vi "emi_Set Application version from Constant.vi"(0 "VI with revision number(this vI)":refnum<vi>, 7 "Version Info in":T1={"Name"="Default Name", "Major"=0, "Minor"=0, "Fix"=0, "Build"=0, "Type"=enum."Alfa", "Dev"=FALSE, "Version Name"="", "Date"=timestamp(0 s since 1904-01-01)} {"Date" format="%<%y%m%d>T"}, 11 "error in (no error)":errorcluster) -> (4 "VI Refnum Out":refnum<vi>, 15 "error out":errorcluster)   [LabVIEW 2011]
doc: "Set the application version information from constant.\n\nWill try to update build and date(on build updated) on version constant on calling diagram\n\nOn error. Sett version anyway, asuming directly from constant. Wil not set version info"
uses:
  Private/emi_Version Info.ctl
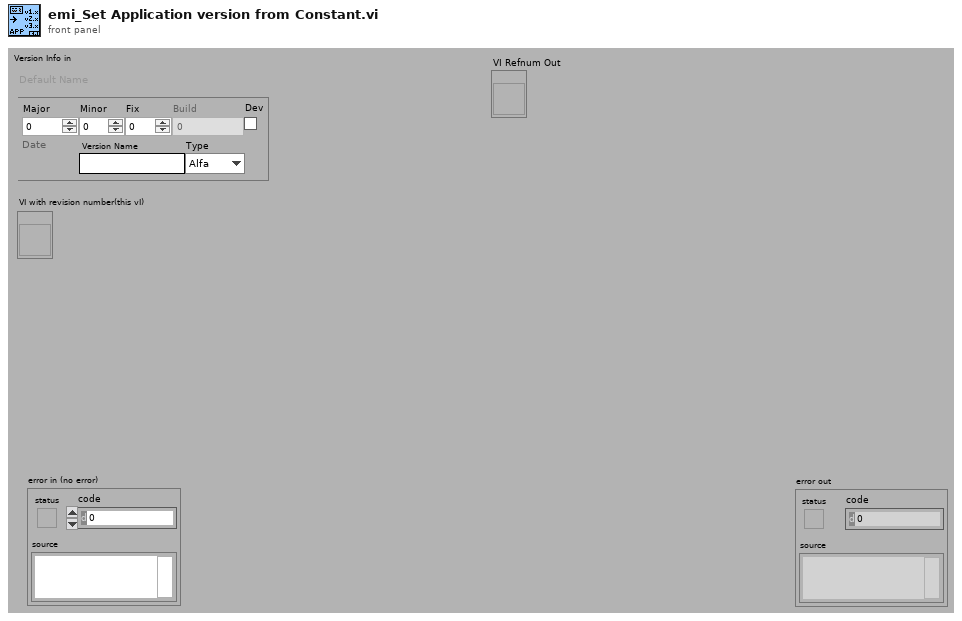
[diagram p1: front panel]
types:
  T1 = typedef "emi_Version Info.ctl" = cluster{"Name":string, "Major":i16, "Minor":i16, "Fix":i16, "Build":i32, "Type":enum16{"Alfa", "Beta", "Stable"}, "Dev":bool, "Version Name":string, "Date":timestamp}
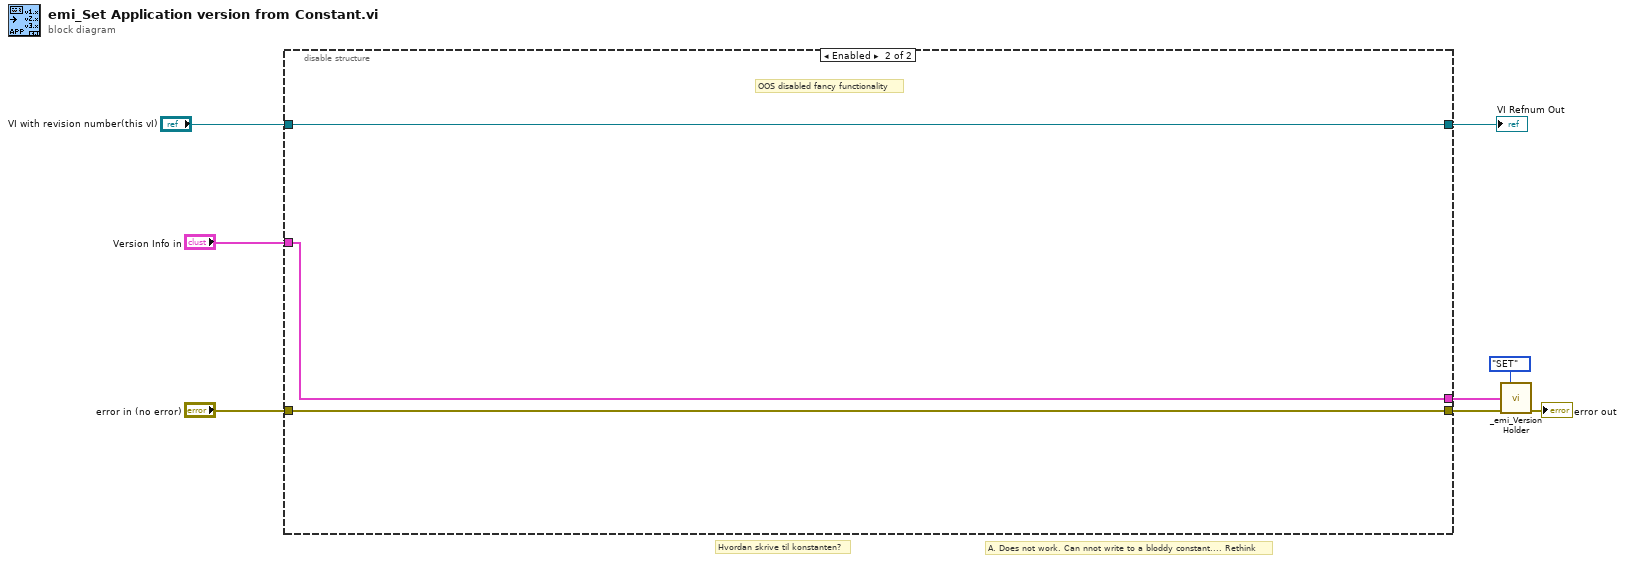
[diagram p0: block diagram]
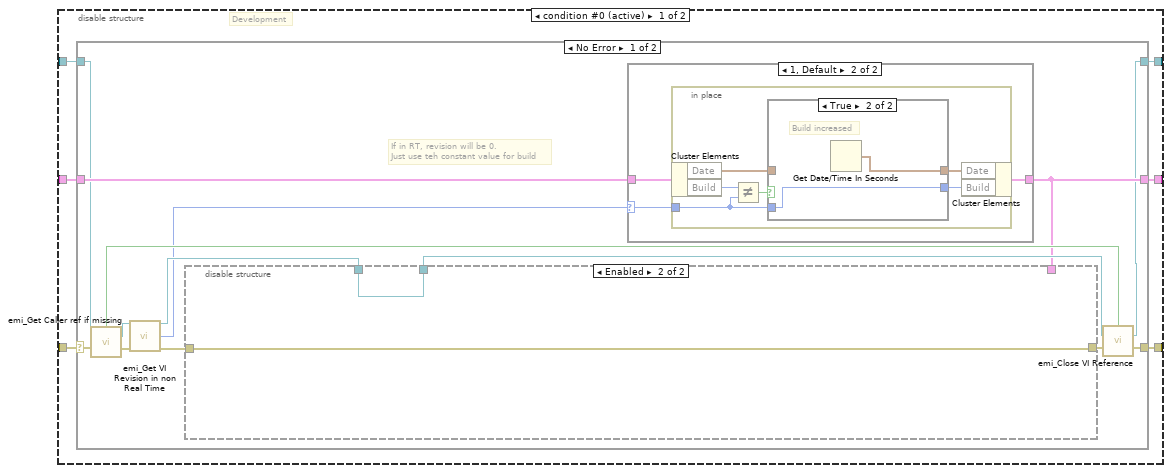
[diagram p3: hidden frame]
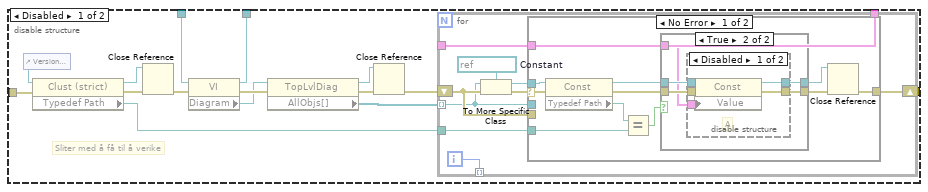
[diagram p6: hidden frame]
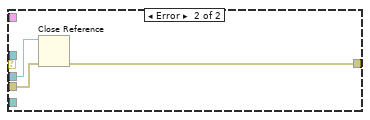
[diagram p9: hidden frame]
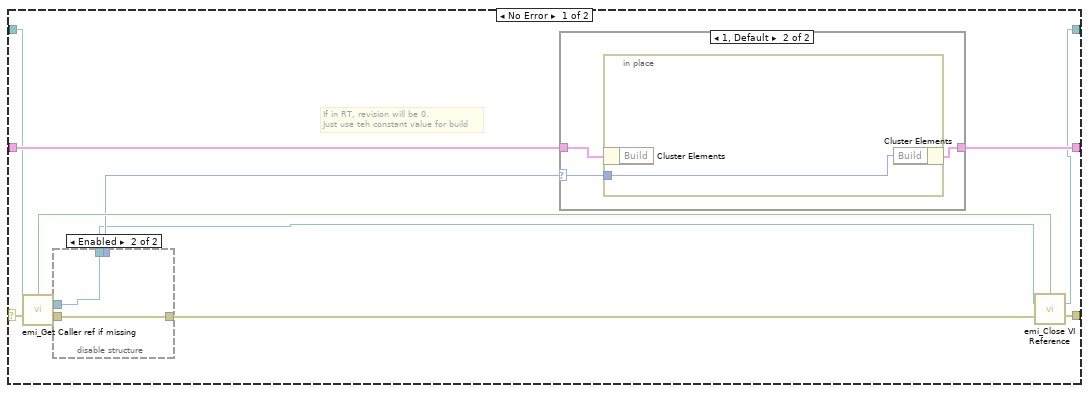
[diagram p11: hidden frame]
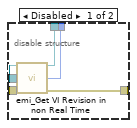
[diagram p12: hidden frame]
diagram:
  # "A. Does not work. Can nnot write to a bloddy constant.... Rethink"
  # "Hvordan skrive til konstanten?"
  n1 = disable-structure shown="Enabled" {
    disable-tunnel: [w14 w141] -> w6
    disable-tunnel: "Version Info in" -> [w13 w141]
    disable-tunnel: "error in (no error)" -> [w12 w140]
    disable-tunnel: [w11 w140] -> w3
    disable-tunnel: "VI with revision number(this vI)" -> [w10 w142]
    disable-tunnel: [w9 w142] -> w1
    frame Disabled {
      n2 = disable-structure shown="RUN_TIME_ENGINE==True, default" {
        disable-tunnel: [w19 w111] -> w14
        disable-tunnel: w13 -> [w20 w112]
        disable-tunnel: w12 -> [w17 w109]
        disable-tunnel: [w18 w110] -> w11
        disable-tunnel: w10 -> [w16 w108]
        disable-tunnel: [w15 w107] -> w9
        frame condition #0 (active) {
          # "Development"
          n3 = case shown="No Error" w17 {
            selector: w17 -> [w26 w106]
            tunnel: w20 -> [w31 w105]
            tunnel: [w24 w105] -> w19
            tunnel: [w30 w106] -> w18
            tunnel: w16 -> [w22 w104]
            tunnel: [w21 w104] -> w15
            frame No Error {
              # "If in RT, revision will be 0.\nJust use teh constant value for build"
              n4 = call "emi_Get Caller ref if missing.vi"("VI Refnum(Calling VI)"=w22, "error in (no error)"=w26) -> ("Ref Generated"=w34:bool, "VI Refnum Out"=w32:refnum<vi>, "error out"=w33:errorcluster)  [unwired: 11 in]
              n5 = call "emi_Get VI Revision in non Real Time.vi"("VI Refnum(This VI)"=w32, "error in (no error)"=w33) -> ("VI Refnum Out"=w28:refnum<vi>, "Vi rev. no"=w23:u32, "error out"=w25:errorcluster)  [unwired: 11 in]
              n6 = case shown="1, Default" w23 {
                selector: w23 -> [_ w36]
                tunnel: w31 -> [w35 w38]
                tunnel: [w35 w37] -> w24
                frame 0 {
                }
                frame 1, Default {
                  n7 = in-place {
                    in-place-border: w36 -> [w39]
                    n8 = in-place-cluster #1(w38) -> ("Date"=w40:timestamp, "Build"=w43:i32)
                    n9 = Not Equal?(x=w43, y=w39) -> (x != y?=w44:bool)
                    n10 = case shown="True" w44 {
                      tunnel: [w45 w47] -> w42
                      tunnel: [w46 w48] -> w41
                      tunnel: w40 -> [w46 _]
                      tunnel: w39 -> [w45 w47]
                      frame False {
                      }
                      frame True {
                        # "Build increased"
                        n11 = Get Date/Time In Seconds() -> (seconds since 1Jan1904=w48:timestamp)
                      }
                    }
                    n12 = in-place-cluster #1("Date"=w41, "Build"=w42) -> (w37:T1)
                  }
                }
              }
              n13 = disable-structure shown="Enabled" {
                disable-tunnel: [w64 w103] -> w29
                disable-tunnel: w28 -> [w61 w103]
                disable-tunnel: [w58 w102] -> w27
                disable-tunnel: w25 -> [w50 w102]
                disable-tunnel: w24 -> [w49 _]
                frame Disabled {
                  # "Sliter med å få til å verike"
                  n14 = control-ref of="Version Info in"() -> (w55:refnum<vi>)
                  n15 = property class="Clust (strict)"(reference=w55, error in=w50) -> (reference out=w54:refnum<vi>, error out=w53:errorcluster, "Typedef Path"=w52:path)
                  n16 = Close Reference(reference=w54, error in (no error)=w53) -> (error out=w51:errorcluster)
                  n17 = property class="VI"(reference=w61, error in=w51) -> (reference out=w64:refnum<vi>, error out=w63:errorcluster, "Diagram"=w59:refnum<vi>)
                  n18 = property class="TopLvlDiag"(reference=w59, error in=w63) -> (reference out=w60:refnum<vi>, error out=w62:errorcluster, "AllObjs[]"=w56:refnum<vi>[])
                  n19 = Close Reference(reference=w60, error in (no error)=w62) -> (error out=w57:errorcluster)
                  n20 = for {
                    tunnel: w56 -> [w66] mode=indexing
                    shift-right: [w69] -> w58
                    shift-left: w57 -> [w67]
                    tunnel: w52 -> [w70]
                    tunnel: w49 -> [w68]
                    tunnel: [w65] -> _ mode=indexing
                    i -> [w65]
                    w73 = refnum<vi> refnum  # Constant
                    n21 = To More Specific Class(target class=w73, reference=w66, error in=w67) -> (specific class reference=w71:refnum<vi>, error out=w72:errorcluster)
                    n22 = case shown="No Error" w72 {
                      selector: w72 -> [w83 _]
                      tunnel: w71 -> [w84 _]
                      tunnel: w70 -> [w81 _]
                      tunnel: [w75 w99] -> w69
                      tunnel: w68 -> [w76 _]
                      tunnel: w67 -> [_ w100]
                      tunnel: w66 -> [_ w101]
                      frame No Error {
                        n23 = property class="Const"(reference=w84, error in=w83) -> (reference out=w78:refnum<vi>, error out=w80:errorcluster, "Typedef Path"=w82:path)
                        n24 = Equal?(x=w82, y=w81) -> (x = y?=w79:bool)
                        n25 = case shown="True" w79 {
                          tunnel: w80 -> [w86 w91]
                          tunnel: w78 -> [w85 w90]
                          tunnel: [w86 w89] -> w77
                          tunnel: w76 -> [_ w87]
                          tunnel: [w85 w88] -> w74
                          frame False {
                          }
                          frame True {
                            n26 = disable-structure shown="Disabled" {
                              disable-tunnel: w91 -> [w96 w97]
                              disable-tunnel: w90 -> [w95 w98]
                              disable-tunnel: [w94 w97] -> w89
                              disable-tunnel: [w93 w98] -> w88
                              disable-tunnel: w87 -> [w92 _]
                              frame Disabled {
                                # "A"
                                n27 = property class="Const"(reference=w95, error in=w96, "Value"=w92) -> (reference out=w93:refnum<vi>, error out=w94:errorcluster)
                              }
                              frame Enabled {
                              }
                            }
                          }
                        }
                        n28 = Close Reference(reference=w74, error in (no error)=w77) -> (error out=w75:errorcluster)
                      }
                      frame Error {
                        n29 = Close Reference(reference=w101, error in (no error)=w100) -> (error out=w99:errorcluster)
                      }
                    }
                  }
                }
                frame Enabled {
                }
              }
              n30 = call "emi_Close VI Reference.vi"("Close ref?(T)"=w34, "VI Refnum"=w29, "error in (no error)"=w27) -> ("VI Refnum Out"=w21:refnum<vi>, "error out"=w30:errorcluster)  [unwired: 11 in]
            }
            frame Error {
            }
          }
        }
        frame condition #1 {
          # "Development"
          n31 = case shown="Error" w109 {
            selector: w109 -> [w119 w139]
            tunnel: w112 -> [w121 w138]
            tunnel: [w118 w138] -> w111
            tunnel: [w120 w139] -> w110
            tunnel: w108 -> [w114 w137]
            tunnel: [w113 w137] -> w107
            frame No Error {
              # "If in RT, revision will be 0.\nJust use teh constant value for build"
              n32 = call "emi_Get Caller ref if missing.vi"("VI Refnum(Calling VI)"=w114, "error in (no error)"=w119) -> ("Ref Generated"=w124:bool, "VI Refnum Out"=w122:refnum<vi>, "error out"=w123:errorcluster)  [unwired: 11 in]
              n33 = disable-structure shown="Enabled" {
                disable-tunnel: w123 -> [w129 w130]
                disable-tunnel: w122 -> [w128 w131]
                disable-tunnel: [w127 _] -> w117
                disable-tunnel: [w126 w131] -> w116
                disable-tunnel: [w125 w130] -> w115
                frame Disabled {
                  n34 = call "emi_Get VI Revision in non Real Time.vi"("VI Refnum(This VI)"=w128, "error in (no error)"=w129) -> ("VI Refnum Out"=w126:refnum<vi>, "Vi rev. no"=w127:u32, "error out"=w125:errorcluster)  [unwired: 11 in]
                }
                frame Enabled {
                }
              }
              n35 = case shown="1, Default" w117 {
                selector: w117 -> [_ w133]
                tunnel: w121 -> [w132 w135]
                tunnel: [w132 w134] -> w118
                frame 0 {
                }
                frame 1, Default {
                  n36 = in-place {
                    in-place-border: w133 -> [w136]
                    n37 = in-place-cluster #2(w135) -> ()  [unwired: 1 out]
                    n38 = in-place-cluster #2("Build"=w136) -> (w134:T1)
                  }
                }
              }
              n39 = call "emi_Close VI Reference.vi"("Close ref?(T)"=w124, "VI Refnum"=w116, "error in (no error)"=w115) -> ("VI Refnum Out"=w113:refnum<vi>, "error out"=w120:errorcluster)  [unwired: 11 in]
            }
            frame Error {
            }
          }
        }
      }
    }
    frame Enabled {
      # "OOS disabled fancy functionality"
    }
  }
  "VI Refnum Out" <- w1
  n40 = call "_emi_Version Holder.vi"("Action(GET)"=enum16{"GET", "SET"}."SET", "Version Info in"=w6, "error in (no error)"=w3) -> ("error out"=→"error out":errorcluster)  [unwired: 10 in, 2 out]
